vi "TimeInterpVariant_SetMaxTime.vi"(9 "Max Time":dbl, 11 "in TimeInterpVariant":T1) -> (3 "out TimeInterpVariant":T1)   [LabVIEW 2019, in "Trajectory_Library.lvlib"]
doc: "Sets the maximum time period that should be stored in the buffer.\n\nInputs:\n - In TimeInterpVariant -- Input data cluster.\n - Max Time -- Maximum time period to store in the buffer (seconds)\n\nOutputs:\n - Out TimeInterpVariant -- Updated data cluster."
uses:
  Trajectory_Library.lvlib
  TypeDef/TIME_INTERPOLATABLE_VARIANT.ctl
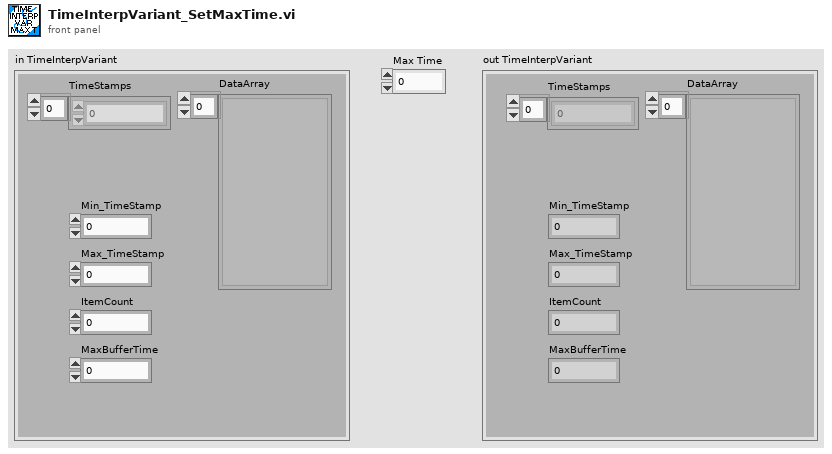
[diagram p1: front panel]
types:
  T1 = typedef "Trajectory_Library.lvlib/TIME_INTERPOLATABLE_VARIANT.ctl" = cluster{"TimeStamps":dbl[], "DataArray":variant[], "Min_TimeStamp":dbl, "Max_TimeStamp":dbl, "ItemCount":i32, "MaxBufferTime":dbl}
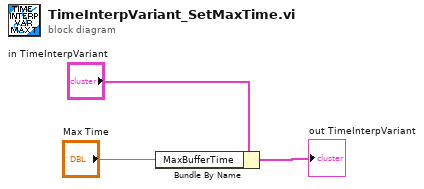
[diagram p0: block diagram]
diagram:
  n1 = Bundle By Name(cluster="in TimeInterpVariant", "MaxBufferTime"="Max Time") -> (→"out TimeInterpVariant":T1)
